vi "CapturaImagenyQR_subVI.vi"() -> (3 "Datos_QR":string)   [LabVIEW 2019]
uses:
  Program Files/National Instruments/LabVIEW 2018/vi.lib/vision/Instrument.llb/QR Code Search Options.ctl
  Program Files/National Instruments/LabVIEW 2018/vi.lib/vision/Instrument.llb/Demodulation Mode.ctl
  Program Files/National Instruments/LabVIEW 2018/vi.lib/vision/Instrument.llb/Cell Sample Size.ctl
  Program Files/National Instruments/LabVIEW 2018/vi.lib/vision/Instrument.llb/Cell Filter Mode.ctl
  Program Files/National Instruments/LabVIEW 2018/vi.lib/vision/Instrument.llb/QR Code Description Options.ctl
  Program Files/National Instruments/LabVIEW 2018/vi.lib/vision/Instrument.llb/Data Matrix Polarity.ctl
  Program Files/National Instruments/LabVIEW 2018/vi.lib/vision/Instrument.llb/QR Code Model Type.ctl
  Program Files/National Instruments/LabVIEW 2018/vi.lib/vision/NI_Vision_Development_Module.lvlib
panel:
  out "path":path=path "C:/Trabajo_Robot/Test Asic Javi_2021/Origen Socket SERVO_PCB_BUENO_v5 (muchos asics)"
  in  "DNVideoX":refnum<k7>(container)
  out "Imagen modificada":T1(plugin-control)
  out "Error":errorcluster
  # "Captura una imagen que guarda como \"CapturaQR.jpg\" en el directorio antes mencionado \n arriba y después accede a esa imagen para leer el código QR (y lo devuelve como un string)."
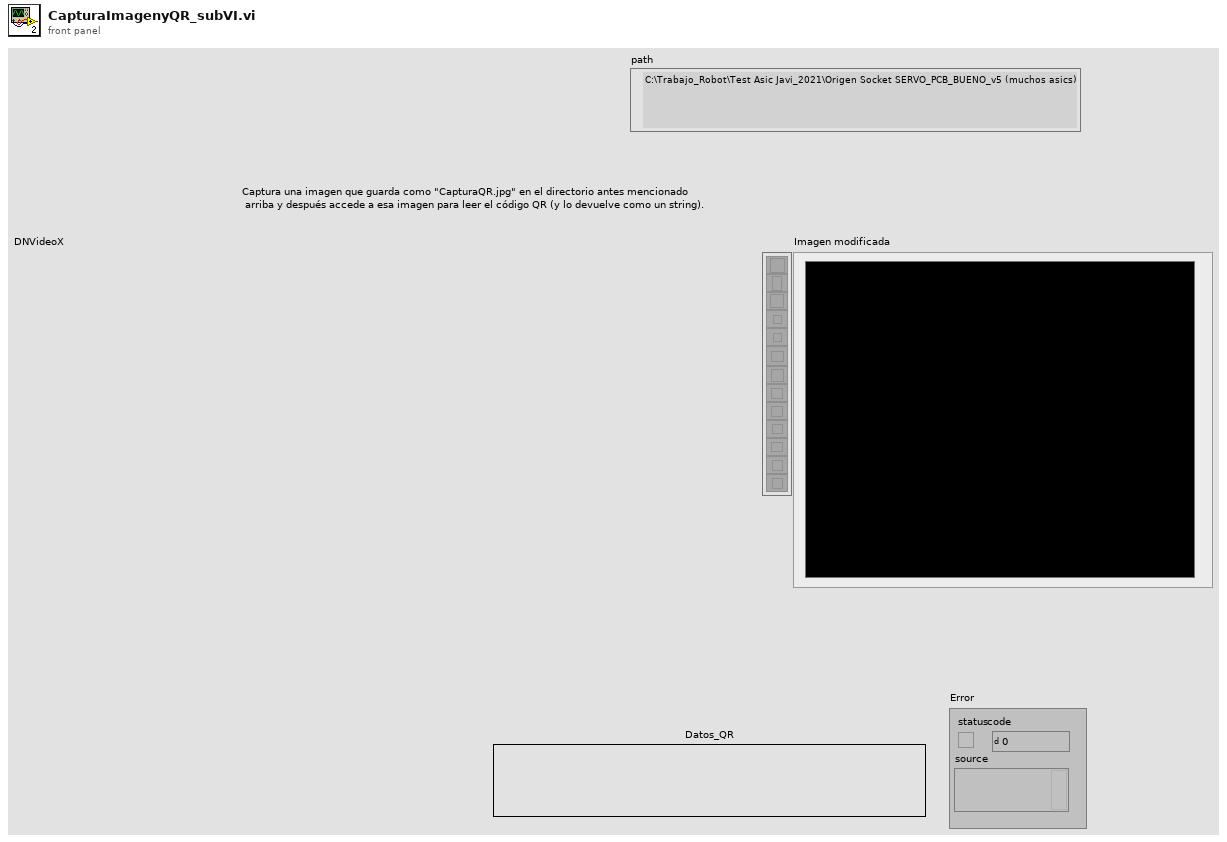
[diagram p1: front panel]
types:
  T1 = typedef "IMAQ Image.ctl" = refnum<image>
  T2 = typedef "QR Code Description Options.ctl" = cluster{"Matrix Size (cells)":i32, "Barcode Polarity":T3, "Mirror Mode":i32, "QR Model":T4}
  T3 = typedef "Data Matrix Polarity.ctl" = i32
  T4 = typedef "QR Code Model Type.ctl" = i32
  T5 = typedef "QR Code Search Options.ctl" = cluster{"Rotation Mode":enum32{"Unlimited", "0 Degrees", "90 Degrees", "180 Degrees", "270 Degrees"}, "Skip Location?":bool, "Edge Threshold":u32, "Demodulation Mode":T6, "Cell Sample Size":T7, "Cell Filter Mode":T8, "Skew Degrees Allowed":u32}
  T6 = typedef "Demodulation Mode.ctl" = i32
  T7 = typedef "Cell Sample Size.ctl" = i32
  T8 = typedef "Cell Filter Mode.ctl" = i32
  T9 = cluster{"Brightness":sgl, "Contrast":sgl, "Gamma":sgl}
  T10 = typedef "QR Code Report.ctl" = cluster{"Found?":bool, "Data":string, "Bounding Box":cluster{"x":sgl, "y":sgl}[], "Errors Corrected":u32, "Dimensions (Rows/Cols)":u32, "Version":u32, "QR Model":T4, "Stream Mode":T11, "Barcode Polarity":T3, "Mirrored?":bool, "Append Stream Position":u32, "Size of Append Stream":u32, "First EAN-128 ID":i32, "First Alternate Language ID":i32, "Append Stream ID":u32, "Minimum Edge Strength":u32, "Demodulation Mode":T6, "Cell Sample Size":T7, "Cell Filter Mode":T8}
  T11 = typedef "QR Code Stream Mode Type.ctl" = i32
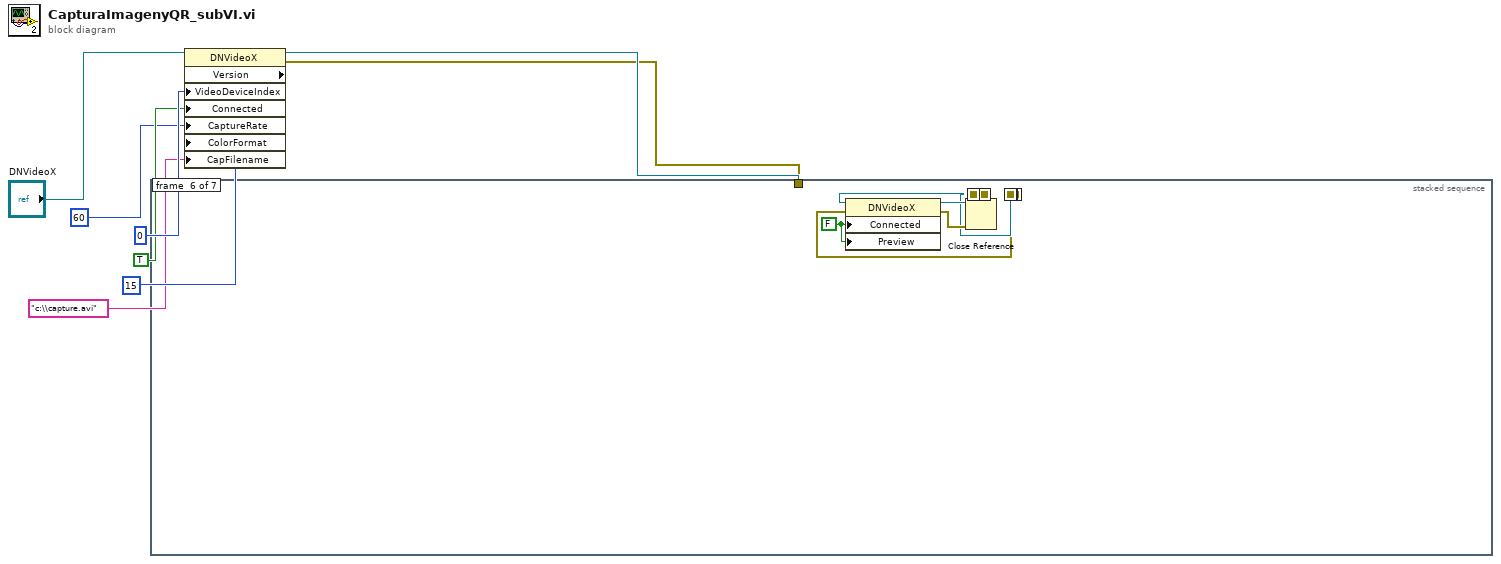
[diagram p0: block diagram]
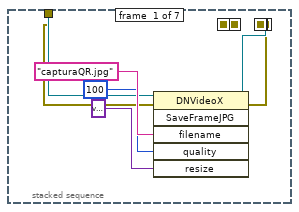
[diagram p2: hidden frame]
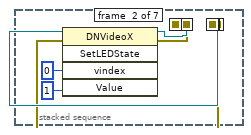
[diagram p3: hidden frame]
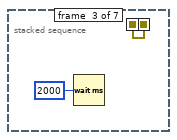
[diagram p4: hidden frame]
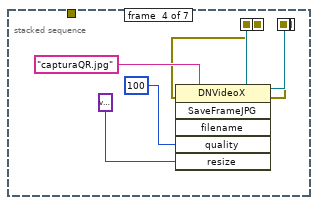
[diagram p5: hidden frame]
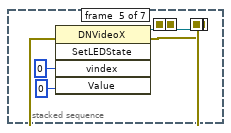
[diagram p6: hidden frame]
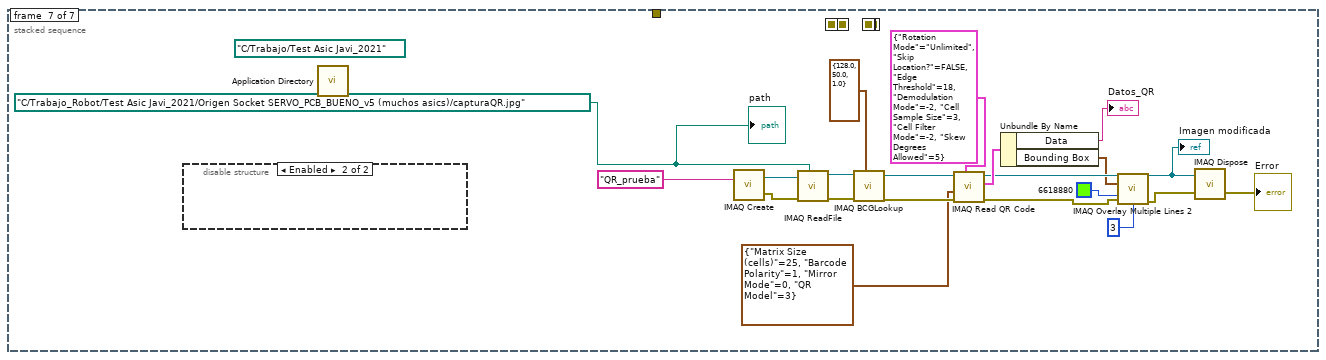
[diagram p7: hidden frame]
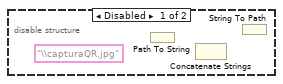
[diagram p8: hidden frame]
diagram:
  n1 = property class="DNVideoX" props=["Version", "VideoDeviceIndex", "Connected", "CaptureRate", "ColorFormat", "CapFilename"](reference="DNVideoX", "VideoDeviceIndex"=0, "Connected"=TRUE, "CaptureRate"=60 ("VideoDeviceIndex"), "ColorFormat"=15 ("VideoDeviceIndex"), "CapFilename"="c:\\capture.avi" ("default name")) -> (reference out=w3:refnum<k7>, error out=w2:errorcluster)  [unwired: 1 in, 1 out]
  n2 = stacked-sequence {
    seq-local: [w10 _ _ _ _ _ _] -> [_ w21 _ _ _ _ _]
    seq-local: [w9 _ _ _ _ _ _] -> [_ w20 _ _ _ _ _]
    seq-local: [_ w19 _ _ _ _ _] -> [_ _ w23 _ _ _ _]
    seq-local: [_ w18 _ _ _ _ _] -> [_ _ w22 _ _ _ _]
    seq-local: [_ _ w23 _ _ _ _] -> [_ _ _ w29 _ _ _]
    seq-local: [_ _ w22 _ _ _ _] -> [_ _ _ w25 _ _ _]
    seq-local: [_ _ _ w27 _ _ _] -> [_ _ _ _ w37 _ _]
    seq-local: [_ _ _ w26 _ _ _] -> [_ _ _ _ w36 _ _]
    seq-local: [_ _ _ _ w35 _ _] -> [_ _ _ _ _ w40 _]
    seq-local: [_ _ _ _ w34 _ _] -> [_ _ _ _ _ w39 _]
    tunnel: w3 -> [w12 _ _ _ _ _ _]
    tunnel: w2 -> [w11 _ _ _ _ _ _]
    frame #0 {
      n3 = invoke class="DNVideoX" method="SaveFrameJPG"(reference=w12, error in=w11, "filename"="capturaQR.jpg", "quality"=100, "resize"=variant) -> (reference out=w10:refnum<k7>, error out=w9:errorcluster)  [unwired: 1 in, 4 out]
    }
    frame #1 {
      n4 = invoke class="DNVideoX" method="SetLEDState"(reference=w21, error in=w20, "vindex"=0, "Value"=1) -> (reference out=w19:refnum<k7>, error out=w18:errorcluster)  [unwired: 1 in, 3 out]
    }
    frame #2 {
      n5 = Wait (ms)(milliseconds to wait=u32 2000) -> ()  [unwired: 1 out]
    }
    frame #3 {
      n6 = invoke class="DNVideoX" method="SaveFrameJPG"(reference=w29, error in=w25, "filename"="capturaQR.jpg", "quality"=100, "resize"=variant) -> (reference out=w27:refnum<k7>, error out=w26:errorcluster)  [unwired: 1 in, 4 out]
    }
    frame #4 {
      n7 = invoke class="DNVideoX" method="SetLEDState"(reference=w37, error in=w36, "vindex"=0, "Value"=0) -> (reference out=w35:refnum<k7>, error out=w34:errorcluster)  [unwired: 1 in, 3 out]
    }
    frame #5 {
      w38 = FALSE ("Connected")
      n8 = property class="DNVideoX"(reference=w40, error in=w39, "Connected"=w38, "Preview"=w38) -> (reference out=w41:refnum<k7>, error out=w42:errorcluster)
      n9 = Close Reference(reference=w41, error in (no error)=w42) -> ()  [unwired: 1 out]
    }
    frame #6 {
      w43 = path "C:/Trabajo_Robot/Test Asic Javi_2021/Origen Socket SERVO_PCB_BUENO_v5 (muchos asics)/capturaQR.jpg" ("path")
      (unwired) path "C:/Trabajo/Test Asic Javi_2021" ("path 2")
      n10 = disable-structure shown="Enabled" {
        frame Disabled {
          (unwired) "\\capturaQR.jpg" ("Image Name")
          n11 = Path To String() -> ()  [unwired: 1 in, 1 out]
          n12 = Concatenate Strings() -> ()  [unwired: 2 in, 1 out]
          n13 = String To Path() -> ()  [unwired: 1 in, 1 out]
        }
        frame Enabled {
        }
      }
      n14 = call <vilib>:"Application Directory.vi"() -> ()  [unwired: 1 out]
      n15 = call "IMAQ Create"("Image Name"="QR_prueba") -> ("New Image"=w51:T1, "error out"=w52:errorcluster)  [unwired: 4 in]
      n16 = call "IMAQ ReadFile"("File Path"=w43, "error in (no error)"=w52, "Image"=w51) -> ("error out"=w61:errorcluster, "Image Out"=w55:T1)  [unwired: 4 in, 3 out]
      n17 = call "IMAQ BCGLookup"("Image Src"=w55, "BCG Values"=T9 {"Brightness"=128.0, "Contrast"=50.0, "Gamma"=1.0}, "error in (no error)"=w61) -> ("Image Dst Out"=w62:T1, "error out"=w63:errorcluster)  [unwired: 4 in]
      n18 = call "IMAQ Read QR Code"("QR Search Options"=T5 {"Rotation Mode"=enum."Unlimited", "Skip Location?"=FALSE, "Edge Threshold"=18, "Demodulation Mode"=-2, "Cell Sample Size"=3, "Cell Filter Mode"=-2, "Skew Degrees Allowed"=5}, "error in (no error)"=w63, "QR Description Options"=T2 {"Matrix Size (cells)"=25, "Barcode Polarity"=1, "Mirror Mode"=0, "QR Model"=3}, "Image"=w62) -> ("error out"=w48:errorcluster, "QR Code Report"=w58:T10, "Image (duplicate)"=w46:T1)  [unwired: 4 in, 1 out]
      n19 = Unbundle By Name(w58) -> ("Data"=→"Datos_QR":string, "Bounding Box"=w45:cluster{"x":sgl, "y":sgl}[])
      n20 = call "IMAQ Overlay Multiple Lines 2"("Image"=w46, "Line End Points"=w45, "Color"=u32 6618880, "error in (no error)"=w48, "Width"=u32 3) -> ("Image Out"=w44:T1, "error out"=w47:errorcluster)  [unwired: 9 in]
      "Imagen modificada" <- w44
      n21 = call "IMAQ Dispose"("Image"=w44, "error in (no error)"=w47) -> ("error out"=→"Error":errorcluster)  [unwired: 4 in]
      "path" <- w43
    }
  }
